vi "Wrap I32 (Zero To Max).vi"(10 "Max":i32, 11 "Value":i32) -> (3 "Wrapped":i32)   [LabVIEW 2018, in "Math.lvlib"]
uses:
  Math.lvlib
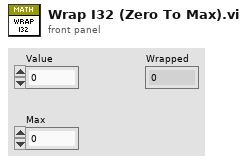
[diagram p1: front panel]
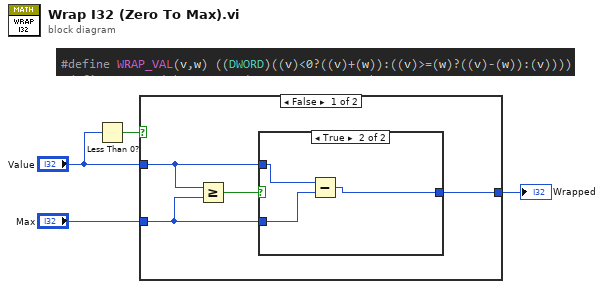
[diagram p0: block diagram]
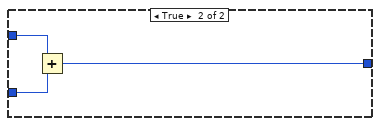
[diagram p3: hidden frame]
diagram:
  n1 = Less Than 0?(x="Value") -> (x < 0?=w4:bool)
  n2 = case shown="False" w4 {
    tunnel: "Value" -> [w8 w15]
    tunnel: "Max" -> [w7 w14]
    tunnel: [w6 w13] -> w1
    frame False {
      n3 = Greater Or Equal?(x=w8, y=w7) -> (x >= y?=w5:bool)
      n4 = case shown="True" w5 {
        tunnel: w8 -> [w9 w12]
        tunnel: w7 -> [_ w11]
        tunnel: [w9 w10] -> w6
        frame False {
        }
        frame True {
          n5 = Subtract(x=w12, y=w11) -> (x-y=w10:i32)
        }
      }
    }
    frame True {
      n6 = Add(x=w15, y=w14) -> (x+y=w13:i32)
    }
  }
  "Wrapped" <- w1
